vi "N02_Case_Structure.vi"() -> ()   [LabVIEW 2023]
panel:
  out "String":string
  out "Numeric":dbl
  in  "Boolean":bool
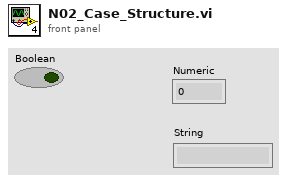
[diagram p1: front panel]
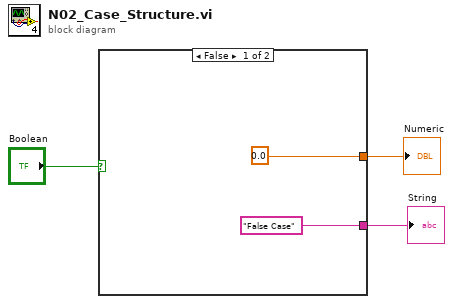
[diagram p0: block diagram]
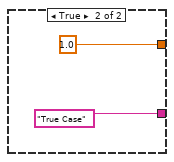
[diagram p2: hidden frame]
diagram:
  n1 = case shown="False" "Boolean" {
    tunnel: [0.0 ("Numeric") 1.0 ("Numeric")] -> w2
    tunnel: ["False Case" ("String") "True Case" ("String")] -> w1
    frame False {
    }
    frame True {
    }
  }
  "Numeric" <- w2
  "String" <- w1
